vi "Save_Zscan.vi"(6 "error in":errorcluster, 8 "Ioca":dbl[](array[numeric]), 9 "Ica":dbl[](array[numeric]), 10 "Ioa":dbl[](array[numeric]), 11 "z (mm)":dbl[](array[numeric])) -> (0 "error out":errorcluster)   [LabVIEW 2010]
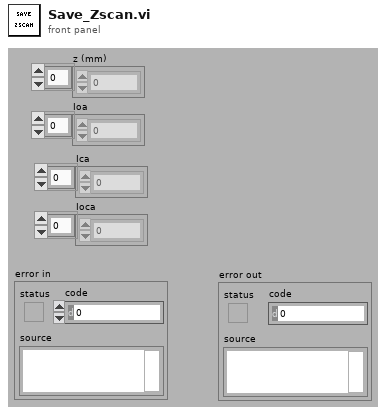
[diagram p1: front panel]
types:
  T1 = enum16{"open", "replace", "create", "open or create", "replace or create", "replace or create with confirmation"}
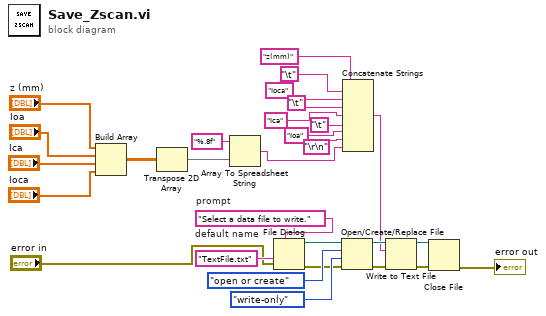
[diagram p0: block diagram]
diagram:
  w23 = "TextFile.txt"  # default name
  w24 = "Select a data file to write."  # prompt
  n1 = Build Array("z (mm)", "Ioa", "Ica", "Ioca") -> (w7:dbl[][])
  n2 = Transpose 2D Array(2D array=w7) -> (transposed array=w19:dbl[][])
  n3 = Array To Spreadsheet String(array=w19, 3:"%.8f") -> (spreadsheet string=w9:string)  [unwired: 1 out]
  n4 = File Dialog(7:w24, 8:"error in", 9:w23) -> (0:w25:errorcluster, 3:w22:path)  [unwired: 6 out]
  n5 = Open/Create/Replace File(file path (use dialog)=w22, error in=w25, operation (0:open)=T1."open or create", access (0:read/write)=enum16{"read/write", "read-only", "write-only"}."write-only") -> (refnum out=w26:refnum<file>, error out=w27:errorcluster)  [unwired: 3 out]
  n6 = Concatenate Strings("z(mm)", "\t", "Ioca", "\t", "Ica", "\t", "Ioa", "\r\n", w9) -> (w8:string)
  n7 = Write to Text File(file (use dialog)=w26, text=w8, error in=w27) -> (refnum out=w20:refnum<file>, error out=w21:errorcluster)  [unwired: 1 in, 1 out]
  n8 = Close File(refnum=w20, error in=w21) -> (error out=→"error out":errorcluster)  [unwired: 1 out]
